vi "File Path Host -- constant.vi"() -> (2 "File Path Control":string)   [LabVIEW 2021, in "TDMS.lvlib"]
uses:
  TDMS.lvlib
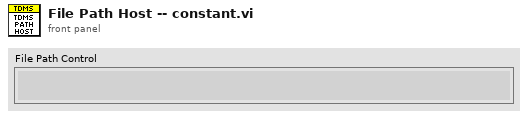
[diagram p1: front panel]
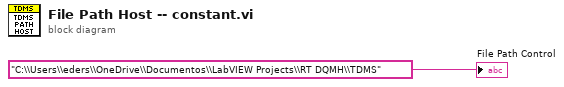
[diagram p0: block diagram]
diagram:
  "File Path Control" <- "C:\\Users\\eders\\OneDrive\\Documentos\\LabVIEW Projects\\RT DQMH\\TDMS"
